vi "CONV String to 2D String.vi"(0 "String":string, 1 "Delimiters (,;)":string=",;") -> (6 "2-D String":string[][](array[string]))   [LabVIEW 2017]
doc: "This routine converts a string list to a 2-D String Array. There should be exactly 2 characters in the Delimiters field. The first is the Column delimiter, and the Second is the Row delimiter.\n\nExample:\n\nString: 1,2,3;4,5,6\nDelimiters: ,;\n\nOutput\n\n1 2 3\n4 5 6"
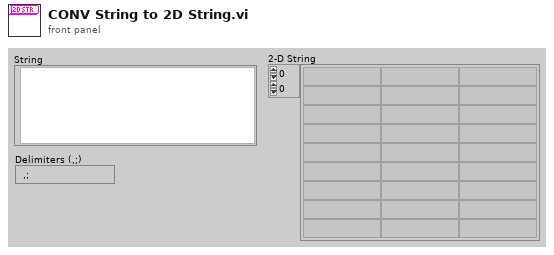
[diagram p1: front panel]
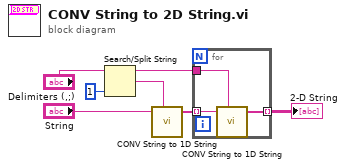
[diagram p0: block diagram]
diagram:
  n1 = Search/Split String(string="Delimiters (,;)", offset (0)=1) -> (substring before match=w3:string, match + rest of string=w4:string)  [unwired: 2 out]
  n2 = call "CONV String to 1D String.vi"("String"="String", "Delimiter (,)"=w4) -> ("1-D String"=w2:string[])  [unwired: 7 out]
  n3 = for {
    tunnel: w3 -> [w9]
    tunnel: w2 -> [w10] mode=indexing
    tunnel: [w8] -> w1 mode=indexing
    n4 = call "CONV String to 1D String.vi"("String"=w10, "Delimiter (,)"=w9) -> ("1-D String"=w8:string[])  [unwired: 7 out]
  }
  "2-D String" <- w1
